vi "HoverButton MakeColot.vi"(11 "Colors [4]":cluster{u32, u32}[](array[cluster])) -> (3 "クラスタ":T1)   [LabVIEW 2014]
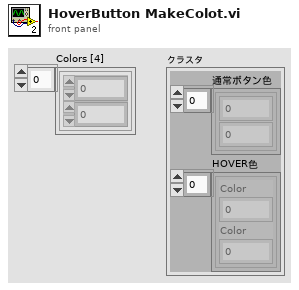
[diagram p1: front panel]
types:
  T1 = cluster{"通常ボタン色":cluster{u32, u32}[], "HOVER色":cluster{"Color":u32, "Color":u32}[]}
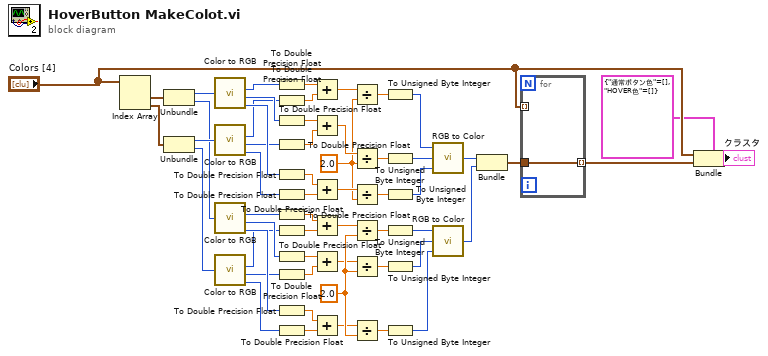
[diagram p0: block diagram]
diagram:
  w50 = 2.0 ("y")
  w16 = 2.0 ("y")
  n1 = Index Array(array="Colors [4]") -> (element #1=w4:cluster{u32, u32}, element #2=w5:cluster{u32, u32})  [unwired: 2 in]
  n2 = Unbundle(w4) -> (w2:u32, w3:u32)
  n3 = Unbundle(w5) -> (w6:u32, w7:u32)
  n4 = call <vilib>:"Color to RGB.vi"("Color"=w2) -> ("R"=w8:u8, "G"=w12:u8, "B"=w15:u8)  [unwired: 1 out]
  n5 = call <vilib>:"Color to RGB.vi"("Color"=w6) -> ("R"=w9:u8, "G"=w13:u8, "B"=w14:u8)  [unwired: 1 out]
  n6 = call <vilib>:"Color to RGB.vi"("Color"=w3) -> ("R"=w30:u8, "G"=w39:u8, "B"=w45:u8)  [unwired: 1 out]
  n7 = call <vilib>:"Color to RGB.vi"("Color"=w7) -> ("R"=w31:u8, "G"=w40:u8, "B"=w46:u8)  [unwired: 1 out]
  n8 = To Double Precision Float(number=w8) -> (double precision float=w21:dbl)
  n9 = To Double Precision Float(number=w9) -> (double precision float=w22:dbl)
  n10 = To Double Precision Float(number=w12) -> (double precision float=w24:dbl)
  n11 = To Double Precision Float(number=w13) -> (double precision float=w25:dbl)
  n12 = To Double Precision Float(number=w15) -> (double precision float=w23:dbl)
  n13 = To Double Precision Float(number=w14) -> (double precision float=w26:dbl)
  n14 = To Double Precision Float(number=w30) -> (double precision float=w33:dbl)
  n15 = To Double Precision Float(number=w31) -> (double precision float=w32:dbl)
  n16 = To Double Precision Float(number=w39) -> (double precision float=w41:dbl)
  n17 = To Double Precision Float(number=w40) -> (double precision float=w42:dbl)
  n18 = To Double Precision Float(number=w45) -> (double precision float=w48:dbl)
  n19 = To Double Precision Float(number=w46) -> (double precision float=w47:dbl)
  n20 = Add(x=w21, y=w22) -> (x+y=w10:dbl)
  n21 = Add(x=w24, y=w25) -> (x+y=w17:dbl)
  n22 = Add(x=w23, y=w26) -> (x+y=w18:dbl)
  n23 = Add(x=w33, y=w32) -> (x+y=w34:dbl)
  n24 = Add(x=w41, y=w42) -> (x+y=w43:dbl)
  n25 = Add(x=w48, y=w47) -> (x+y=w49:dbl)
  n26 = Divide(x=w10, y=w16) -> (x/y=w11:dbl)
  n27 = Divide(x=w17, y=w16) -> (x/y=w19:dbl)
  n28 = Divide(x=w18, y=w16) -> (x/y=w20:dbl)
  n29 = Divide(x=w34, y=w50) -> (x/y=w35:dbl)
  n30 = Divide(x=w43, y=w50) -> (x/y=w44:dbl)
  n31 = Divide(x=w49, y=w50) -> (x/y=w51:dbl)
  n32 = To Unsigned Byte Integer(number=w11) -> (unsigned 8bit integer=w27:u8)
  n33 = To Unsigned Byte Integer(number=w19) -> (unsigned 8bit integer=w28:u8)
  n34 = To Unsigned Byte Integer(number=w20) -> (unsigned 8bit integer=w29:u8)
  n35 = To Unsigned Byte Integer(number=w35) -> (unsigned 8bit integer=w36:u8)
  n36 = To Unsigned Byte Integer(number=w44) -> (unsigned 8bit integer=w37:u8)
  n37 = To Unsigned Byte Integer(number=w51) -> (unsigned 8bit integer=w38:u8)
  n38 = call <vilib>:"RGB to Color.vi"("B"=w29, "G"=w28, "R"=w27) -> ("Color"=w52:u32)
  n39 = call <vilib>:"RGB to Color.vi"("B"=w38, "G"=w37, "R"=w36) -> ("Color"=w53:u32)
  n40 = Bundle("Color"=w52, "Color"=w53) -> (w54:cluster{"Color":u32, "Color":u32})  [unwired: 1 in]
  n41 = for {
    tunnel: w54 -> [w58]
    tunnel: "Colors [4]" -> [_] mode=indexing
    tunnel: [w58] -> w55 mode=indexing
  }
  n42 = Bundle(cluster=T1 {"通常ボタン色"=[], "HOVER色"=[]} ("クラスタ"), "通常ボタン色"="Colors [4]", "HOVER色"=w55) -> (→"クラスタ":T1)
